vi "Main Control.vi"() -> ()   [LabVIEW 2016]
uses:
  Main/main.lvlib
  Main/main control case.ctl
  Main/beamline selection.ctl
  control vi/main/save load/saveload.ctl
  Main/tool selection.ctl
panel:
  out "run vis Error":errorcluster[][](array[cluster])
  in  "change sample":bool
  in  "sample number":i32=1 min=1 max=64 step=1
  in  "pop? upper":bool
  in  "error in":errorcluster
  out "error out":errorcluster
  in  "Upper Panel Display":T1 items=["Calulated values", "Scale", "Currents", "Injector magnet", "Detector settings", "Terminal Voltage", "Source BPM", "Change Foil", "Vacuum", "Flat Top", "zero values", "Terminal Control", "scan injector"]
  in  "pop?":bool
  in  "stop":bool
  in  "Lower Panel Display":T2 items=["Source A", "Source B", "Low End", "High End", "Transmission", "R30", "R45"]
  in  "Cluster":T3
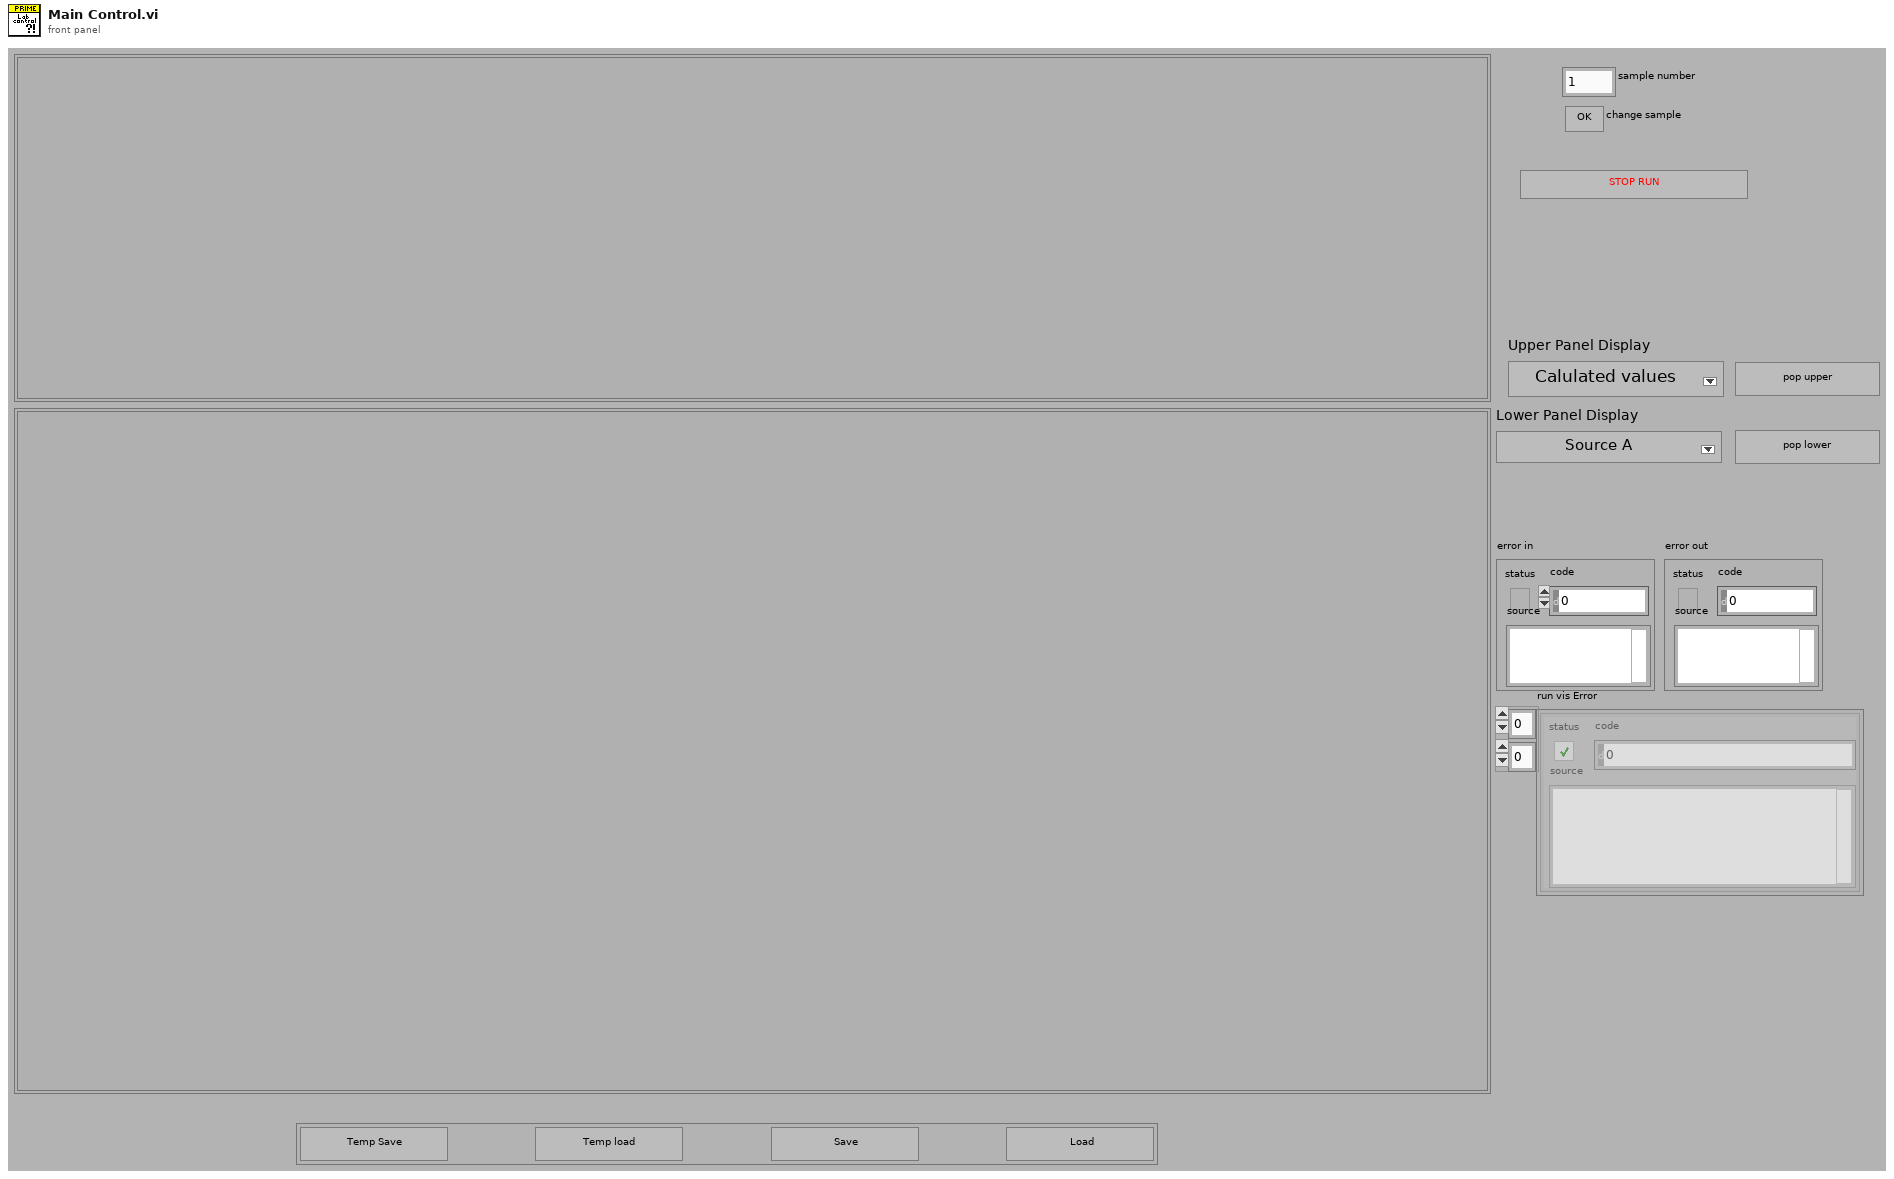
[diagram p1: front panel]
types:
  T1 = typedef "main.lvlib/tool selection.ctl" = u16
  T2 = typedef "main.lvlib/beamline selection.ctl" = u16
  T3 = typedef "main.lvlib/saveload.ctl" = cluster{"OK Button":bool, "OK Button 2":bool, "OK Button 3":bool, "OK Button 4":bool}
  T4 = typedef "main.lvlib/main control case.ctl" = enum16{"Wait", "change beamline section", "change upper section", "Pop vi", "Save vi", "Stop", "upper pop up"}
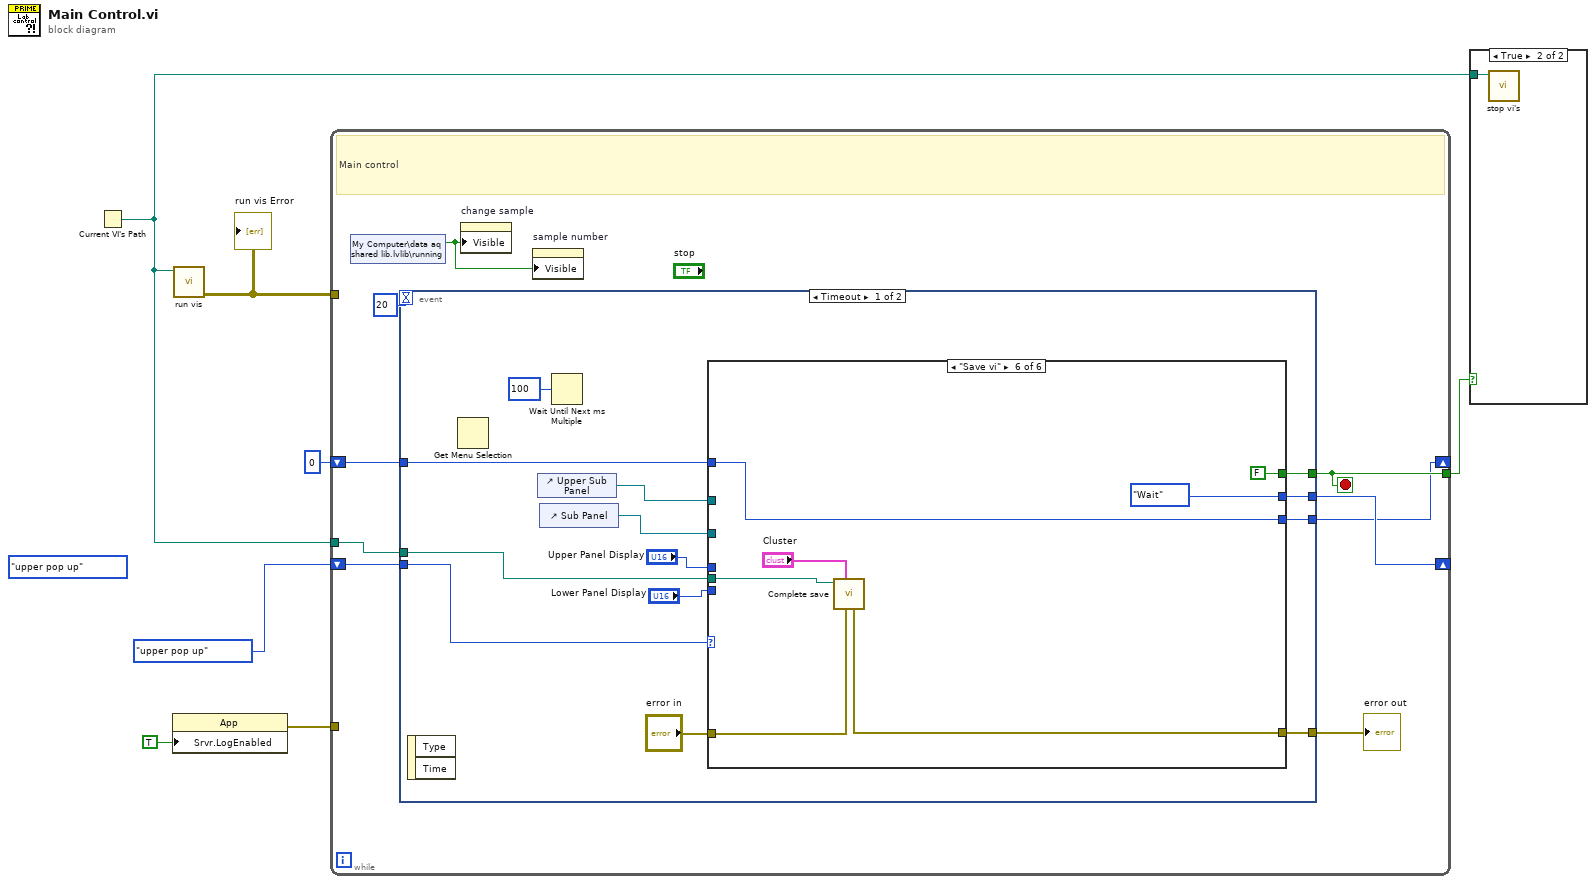
[diagram p0: block diagram]
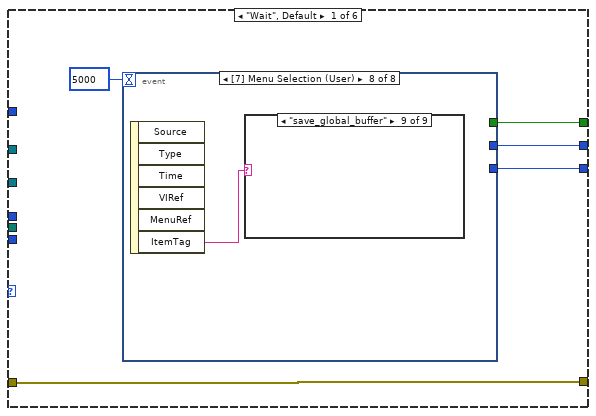
[diagram p3: hidden frame]
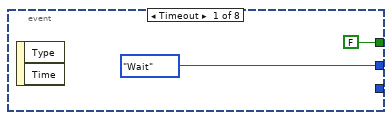
[diagram p4: hidden frame]
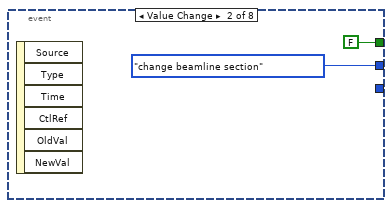
[diagram p5: hidden frame]
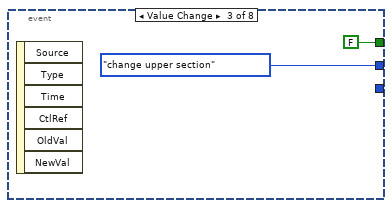
[diagram p6: hidden frame]
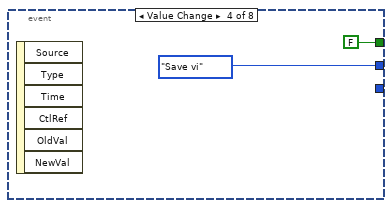
[diagram p7: hidden frame]
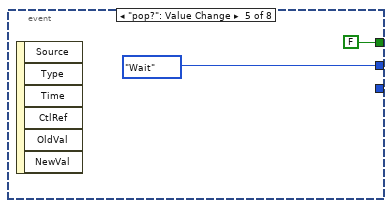
[diagram p8: hidden frame]
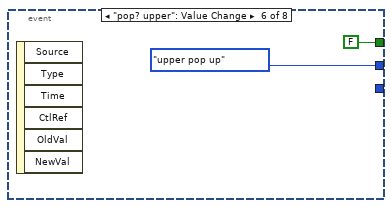
[diagram p9: hidden frame]
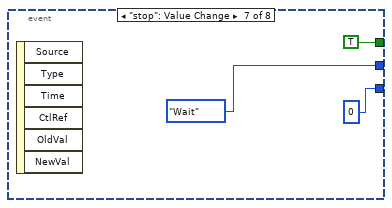
[diagram p10: hidden frame]
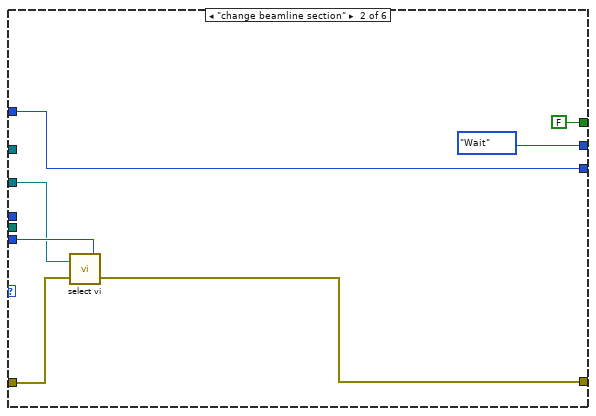
[diagram p19: hidden frame]
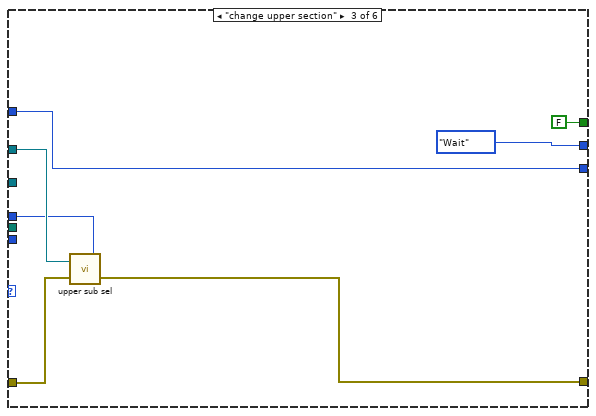
[diagram p20: hidden frame]
diagram:
  (unwired) main_control_case."upper pop up" ("Ring")
  n1 = Current VI's Path() -> (path=w4:path)
  n2 = property class="App"("Srvr.LogEnabled"=TRUE ("Server:Logging Enabled")) -> (error out=w2:errorcluster)  [unwired: 2 in, 1 out]
  n3 = call "run vis.vi"("home path"=w4) -> ("run vis Error"=w5:errorcluster[][])  [unwired: 1 in, 9 out]
  "run vis Error" <- w5
  n4 = while {
    tunnel: [w14] -> w7
    shift-right: [w16] -> _
    shift-left: main_control_case."upper pop up" ("main control case") -> [w15]
    shift-right: [w13] -> _
    shift-left: 0 ("index of element") -> [w12]
    tunnel: w5 -> [_]
    tunnel: w4 -> [w10]
    tunnel: w2 -> [_]
    stop <- w14 stop-if-true
    # "Main control"
    n5 = shared-variable "My Computer\\data aq shared lib.lvlib\\running"() -> (w8:bool)  [unwired: 1 in, 1 out]
    n6 = event shown="[0] Timeout" {
      selector: _ -> [_ _]
      dyn-events: _ -> [_ _]
      timeout: 20 -> [_ _]
      tunnel: [w28 main_control_case."Wait" ("main control case")] -> w16
      tunnel: w15 -> [w27 _]
      tunnel: [w26 _] -> w14
      tunnel: [w21 _] -> w13
      tunnel: w12 -> [w20 _]
      tunnel: w10 -> [w18 _]
      tunnel: [w17 _] -> w9
      event Timeout {
        n7 = event-data() -> ()  [unwired: 1 in, 2 out]
        n8 = Get Menu Selection() -> ()  [unwired: 4 in, 5 out]
        n9 = control-ref of="Upper Sub Panel"() -> (w22:refnum<vi>)
        n10 = control-ref of="Sub Panel"() -> (w24:refnum<vi>)
        n11 = Wait Until Next ms Multiple(millisecond multiple=u32 100) -> ()  [unwired: 1 out]
        n12 = case shown="\"Save vi\"" w27 {
          tunnel: [w34 main_control_case."Wait" ("main control case") main_control_case."Wait" ("main control case") main_control_case."Wait" ("main control case") main_control_case."Wait" ("main control case") main_control_case."Wait" ("main control case")] -> w28
          tunnel: [w33 FALSE ("stop") FALSE ("stop") FALSE ("stop") FALSE ("stop") FALSE ("stop")] -> w26
          tunnel: "Lower Panel Display" -> [_ w57 _ w70 _ _]
          tunnel: w24 -> [_ w56 _ w71 _ _]
          tunnel: "Upper Panel Display" -> [_ _ w63 _ w74 _]
          tunnel: w22 -> [_ _ w64 _ w75 _]
          tunnel: [w31 w54 w61 w68 w79 w85] -> w21
          tunnel: w20 -> [_ w54 w61 w68 w79 w85]
          tunnel: [w30 w53 w60 w67 w78 w83] -> w17
          tunnel: "error in" -> [w30 w52 w59 w66 w77 w84]
          tunnel: w18 -> [_ _ _ _ _ w82]
          frame "Wait", Default {
            n13 = event shown="[7] Menu Selection (User)" {
              selector: _ -> [_ _ _ _ _ _ _ _]
              dyn-events: _ -> [_ _ _ _ _ _ _ _]
              timeout: 5000 -> [_ _ _ _ _ _ _ _]
              tunnel: [main_control_case."Wait" ("main control case") main_control_case."change beamline section" ("main control case") main_control_case."change upper section" ("main control case") main_control_case."Save vi" ("main control case") main_control_case."Wait" ("main control case") main_control_case."upper pop up" ("main control case") main_control_case."Wait" ("main control case") _] -> w34
              tunnel: [FALSE ("stop") FALSE ("stop") FALSE ("stop") FALSE ("stop") FALSE ("stop") FALSE ("stop") TRUE ("stop") _] -> w33
              tunnel: [_ _ _ _ _ _ 0 ("t") _] -> w31
              event Timeout {
                n14 = event-data() -> ()  [unwired: 3 out]
              }
              event Value Change {
                n15 = event-data() -> ()  [unwired: 7 out]
              }
              event Value Change {
                n16 = event-data() -> ()  [unwired: 7 out]
              }
              event Value Change {
                n17 = event-data() -> ()  [unwired: 7 out]
              }
              event "pop?": Value Change {
                n18 = event-data() -> ()  [unwired: 7 out]
              }
              event "pop? upper": Value Change {
                n19 = event-data() -> ()  [unwired: 7 out]
              }
              event "stop": Value Change {
                n20 = event-data() -> ()  [unwired: 7 out]
              }
              event Menu Selection (User) {
                n21 = event-data() -> ("ItemTag"=w50:string)  [unwired: 6 out]
                n22 = case shown="\"save_global_buffer\"" w50 {
                  frame "False", Default {
                  }
                  frame "load_local_file" {
                  }
                  frame "load_local_buffer" {
                  }
                  frame "load_global_file" {
                  }
                  frame "load_global_buffer" {
                  }
                  frame "save_local_file" {
                  }
                  frame "save_local_buffer" {
                  }
                  frame "save_global_file" {
                  }
                  frame "save_global_buffer" {
                  }
                }
              }
            }
          }
          frame "change beamline section" {
            n23 = call "select vi.vi"("Beamline Section"=w57, "error in (no error)"=w52, "reference"=w56) -> ("error out"=w53:errorcluster)
          }
          frame "change upper section" {
            n24 = call "upper sub sel.vi"("Ring"=w63, "error in (no error)"=w59, "SubPnl Refnum"=w64) -> ("error out"=w60:errorcluster)
          }
          frame "Pop vi" {
            n25 = call "pop vi.vi"("pop vi"="pop?", "error in (no error)"=w66, "Beamline Section"=w70, "Sub Panel"=w71) -> ("error out"=w67:errorcluster)
          }
          frame "upper pop up" {
            n26 = call "upper pop.vi"("pop vi"="pop? upper", "error in (no error)"=w77, "Ring"=w74, "Sub Panel"=w75) -> ("error out"=w78:errorcluster)
          }
          frame "Save vi" {
            n27 = call "Complete save.vi"("error in"=w84, "save/load cluster"="Cluster", "home path"=w82) -> ("error out 3"=w83:errorcluster)  [unwired: 8 in]
          }
        }
      }
      event "change sample": Value Change {
        n28 = event-data() -> ()  [unwired: 1 in, 5 out]
        n29 = shared-variable "My Computer\\sc shared var.lvlib\\change sample"("change sample") -> ()  [unwired: 1 in, 1 out]
        n30 = shared-variable "My Computer\\sc shared var.lvlib\\sample number"("sample number") -> ()  [unwired: 1 in, 1 out]
      }
    }
    "error out" <- w9
    n31 = property on="change sample" class="Bool"("Visible"=w8) -> ()  [unwired: 2 in, 2 out]
    n32 = property on="sample number" class="DigNum (strict)"("Visible"=w8) -> ()  [unwired: 2 in, 2 out]
  }
  n33 = case shown="True" w7 {
    tunnel: w4 -> [_ w91]
    frame False {
    }
    frame True {
      n34 = call "stop vi's.vi"("home path"=w91) -> ()  [unwired: 1 in, 10 out]
    }
  }
